vi "Main.vi"() -> ()   [LabVIEW 2019]
panel:
  out "wait mS":u16=250
  out "Board":picture
  out "Next Piece":picture
  out "Rows Cleared":u16
  out "Score":u32
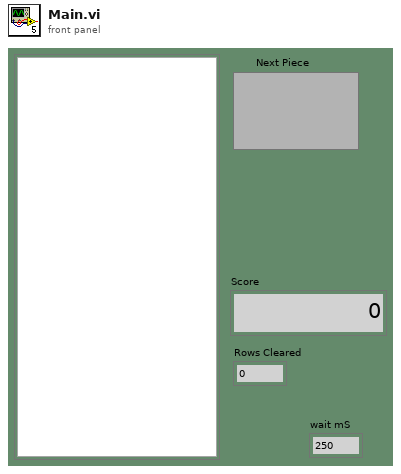
[diagram p1: front panel]
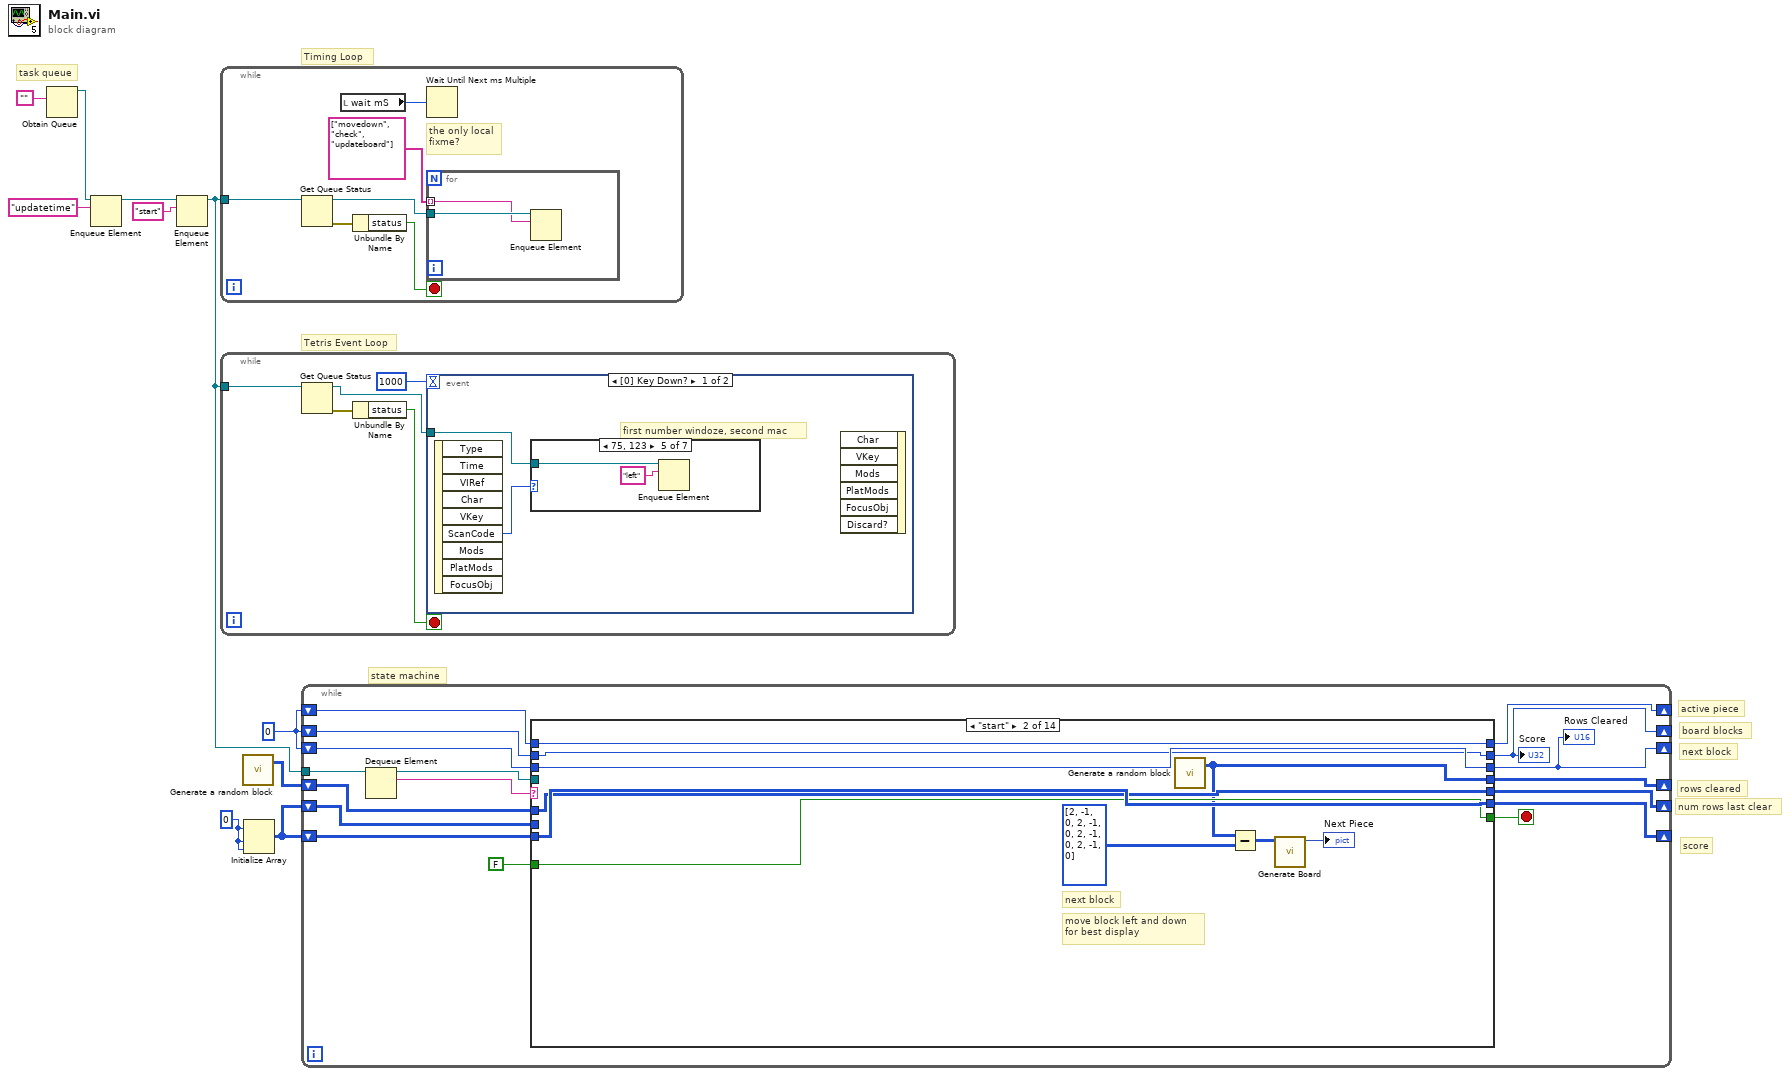
[diagram p0: block diagram]
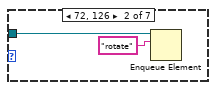
[diagram p3: hidden frame]
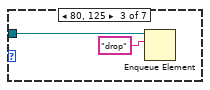
[diagram p4: hidden frame]
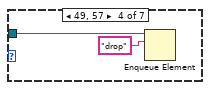
[diagram p5: hidden frame]
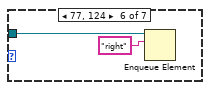
[diagram p6: hidden frame]
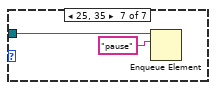
[diagram p7: hidden frame]
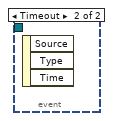
[diagram p8: hidden frame]
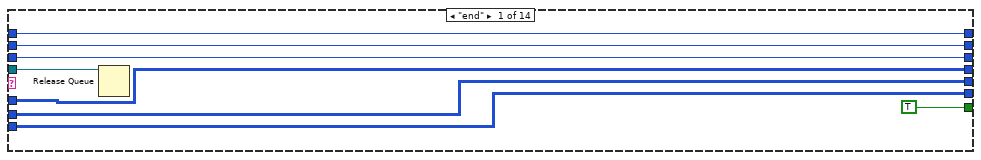
[diagram p9: hidden frame]
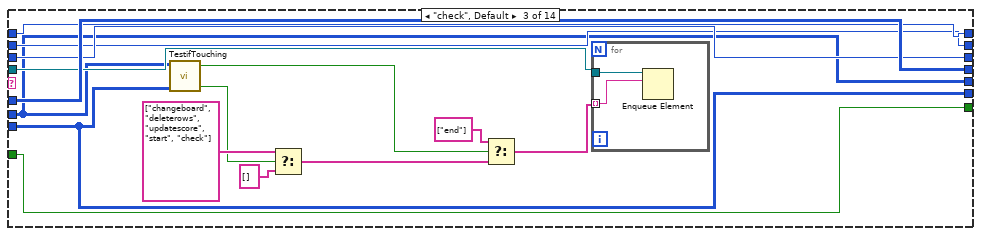
[diagram p10: hidden frame]
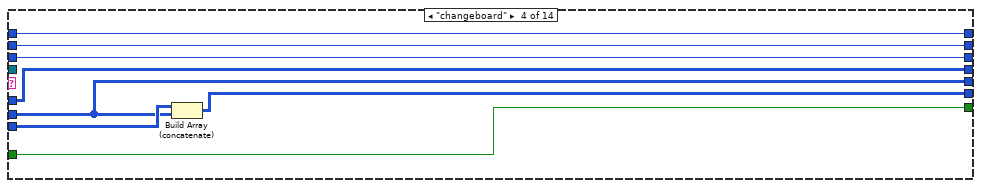
[diagram p11: hidden frame]
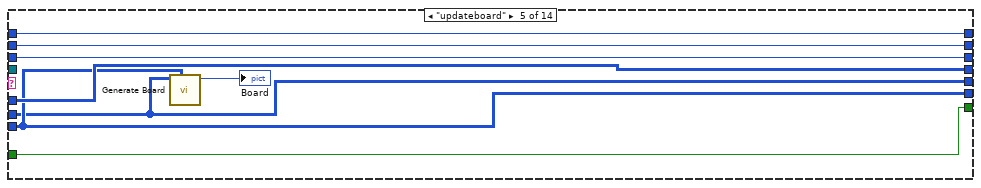
[diagram p12: hidden frame]
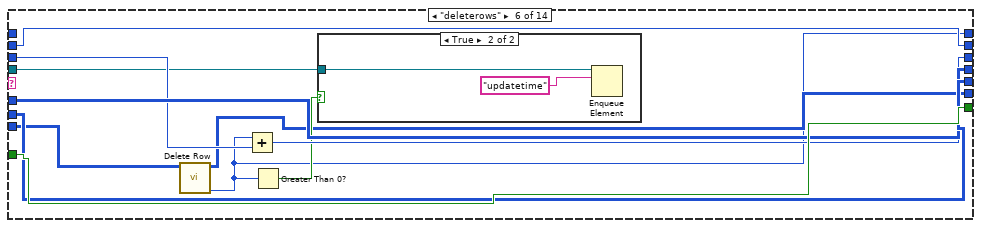
[diagram p13: hidden frame]
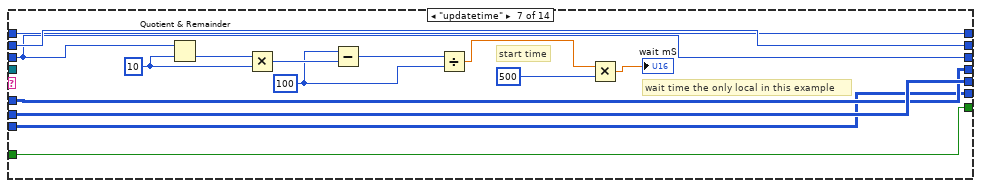
[diagram p15: hidden frame]
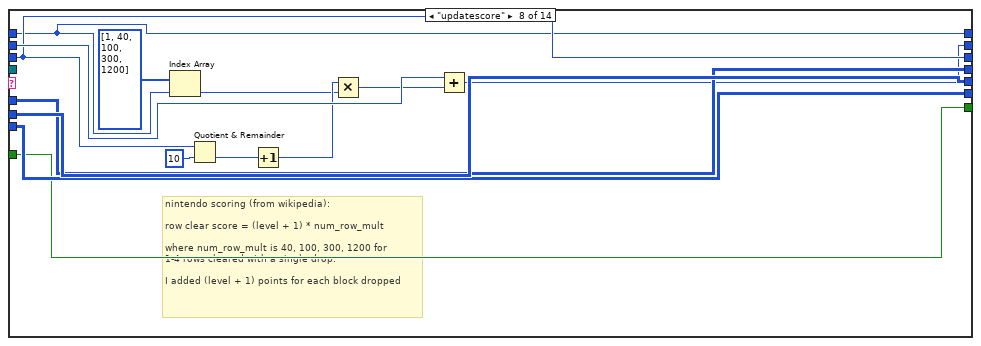
[diagram p16: hidden frame]
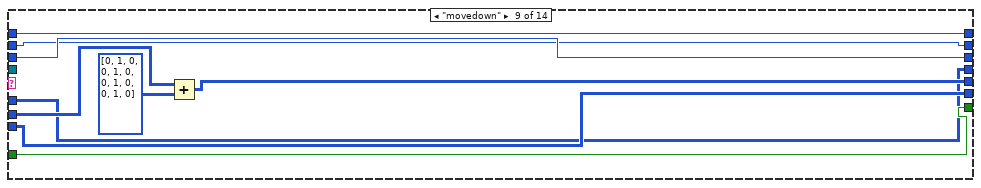
[diagram p17: hidden frame]
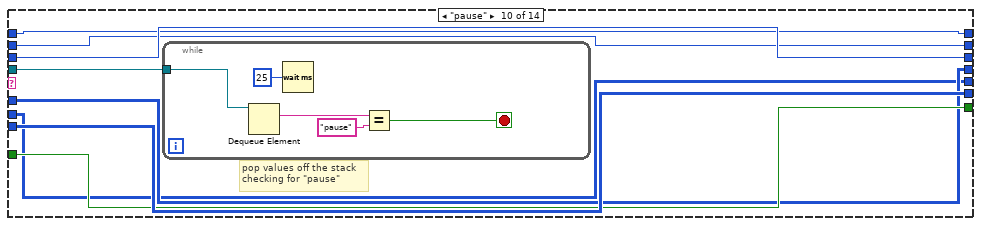
[diagram p18: hidden frame]
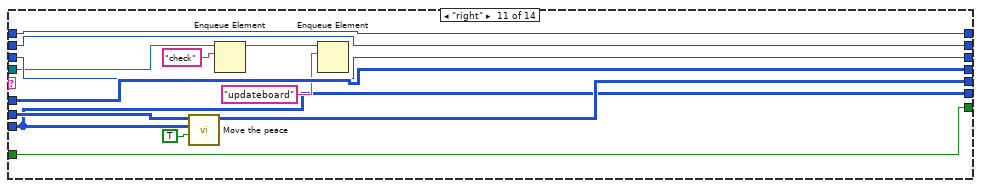
[diagram p19: hidden frame]
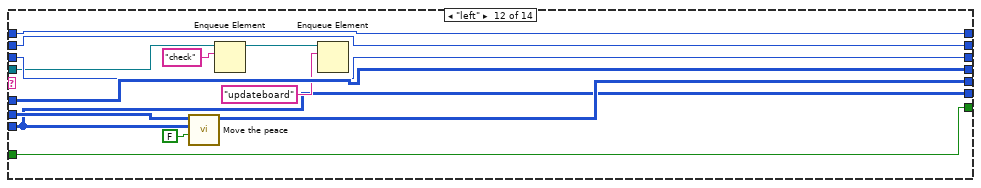
[diagram p20: hidden frame]
diagram:
  w2 = 0
  w10 = 0
  # "task queue"
  # "num rows last clear"
  # "score"
  # "rows cleared"
  # "Timing Loop"
  # "Tetris Event Loop"
  # "state machine"
  # "next block"
  # "board blocks"
  # "active piece"
  n1 = Obtain Queue(element data type="") -> (queue out=w8:refnum<queue>)  [unwired: 4 in, 2 out]
  n2 = Enqueue Element(queue=w8, element="updatetime") -> (queue out=w5:refnum<queue>)  [unwired: 2 in, 2 out]
  n3 = Enqueue Element(queue=w5, element="start") -> (queue out=w4:refnum<queue>)  [unwired: 2 in, 2 out]
  n4 = while {
    tunnel: w4 -> [w12]
    stop <- w13 stop-if-true
    # "the only local\nfixme?"
    n5 = Get Queue Status(queue=w12) -> (queue out=w11:refnum<queue>, error out=w14:errorcluster)  [unwired: 2 in, 6 out]
    n6 = local read "wait mS"() -> (w15:u16)
    n7 = Unbundle By Name(w14) -> ("status"=w13:bool)
    n8 = Wait Until Next ms Multiple(millisecond multiple=w15) -> ()  [unwired: 1 out]
    n9 = for {
      tunnel: w11 -> [w18]
      tunnel: string[] ["movedown", "check", "updateboard"] -> [w17] mode=indexing
      n10 = Enqueue Element(queue=w18, element=w17) -> ()  [unwired: 2 in, 3 out]
    }
  }
  n11 = while {
    tunnel: w4 -> [w20]
    stop <- w21 stop-if-true
    n12 = Get Queue Status(queue=w20) -> (queue out=w19:refnum<queue>, error out=w22:errorcluster)  [unwired: 2 in, 6 out]
    n13 = Unbundle By Name(w22) -> ("status"=w21:bool)
    n14 = event shown="[0] Key Down?" {
      selector: _ -> [_ _]
      dyn-events: _ -> [_ _]
      timeout: 1000 -> [_ _]
      tunnel: w19 -> [w24 _]
      event Key Down? {
        # "first number windoze, second mac"
        n15 = event-data() -> ("ScanCode"=w25:i16)  [unwired: 1 in, 8 out]
        n16 = case shown="75, 123" w25 {
          tunnel: w24 -> [_ w27 w29 w31 w33 w35 w37]
          frame 0, Default {
          }
          frame 72, 126 {
            n17 = Enqueue Element(queue=w27, element="rotate") -> ()  [unwired: 2 in, 3 out]
          }
          frame 80, 125 {
            n18 = Enqueue Element(queue=w29, element="drop") -> ()  [unwired: 2 in, 3 out]
          }
          frame 49, 57 {
            n19 = Enqueue Element(queue=w31, element="drop") -> ()  [unwired: 2 in, 3 out]
          }
          frame 75, 123 {
            n20 = Enqueue Element(queue=w33, element="left") -> ()  [unwired: 2 in, 3 out]
          }
          frame 77, 124 {
            n21 = Enqueue Element(queue=w35, element="right") -> ()  [unwired: 2 in, 3 out]
          }
          frame 25, 35 {
            n22 = Enqueue Element(queue=w37, element="pause") -> ()  [unwired: 2 in, 3 out]
          }
        }
        n23 = event-data() -> ()  [unwired: 7 in, 1 out]
      }
      event Timeout {
        n24 = event-data() -> ()  [unwired: 1 in, 3 out]
      }
    }
  }
  n25 = call "Generate a random block.vi"() -> ("Block Array"=w1:u8[][])  [unwired: 3 in]
  n26 = Initialize Array(w10, w10, w10) -> (w6:i32[][])
  n27 = while {
    shift-right: [w44] -> _
    shift-left: w6 -> [w52]
    shift-right: [w45] -> _
    shift-left: w6 -> [w51]
    shift-right: [w49] -> _
    shift-left: w1 -> [w50]
    tunnel: w4 -> [w48]
    shift-right: [w42] -> _
    shift-left: w2 -> [w43]
    shift-right: [w39] -> _
    shift-left: w2 -> [w40]
    shift-right: [w38] -> _
    shift-left: w2 -> [w41]
    stop <- w53 stop-if-true
    n28 = Dequeue Element(queue=w48) -> (queue out=w47:refnum<queue>, element=w46:string)  [unwired: 2 in, 2 out]
    n29 = case shown="\"start\"" w46 {
      tunnel: FALSE -> [_ w66 w87 w97 w105 w116 w133 w145 w152 w163 w182 w195 w207 w219]
      tunnel: [TRUE w66 w87 w97 w105 w116 w133 w145 w152 w163 w182 w195 w207 w219] -> w53
      tunnel: [w61 w71 w76 w95 w98 w115 w132 w147 w153 w161 w172 w185 w196 w210] -> w44
      tunnel: w52 -> [w61 _ w76 w95 w98 w115 w132 w147 w155 w161 w173 w186 w198 w210]
      tunnel: w51 -> [w60 w72 w75 w96 w99 w108 w130 w146 w156 w164 w171 w184 w197 w209]
      tunnel: [w60 w72 w75 w94 w99 w107 w130 w146 w156 w164 w171 w184 w197 w209] -> w45
      tunnel: w50 -> [w59 w71 w85 w93 w104 w114 w131 w144 w151 w162 w181 w194 w206 w218]
      tunnel: [w59 w65 w85 w93 w104 w114 w131 w144 w151 w162 w181 w194 w206 w218] -> w49
      tunnel: w47 -> [w55 _ w84 _ _ w111 _ _ _ w160 w176 w189 w199 w215]
      tunnel: [w58 w69 w79 w92 w103 w112 w128 w141 w150 w159 w180 w193 w205 w213] -> w42
      tunnel: w43 -> [w58 w69 w79 w92 w103 w113 w128 w141 w150 w159 w180 w193 w205 w213]
      tunnel: [w57 w68 w78 w91 w102 w106 w127 w139 w149 w158 w179 w192 w204 w212] -> w39
      tunnel: [w56 w67 w77 w90 w101 w110 w129 w135 w148 w157 w178 w191 w203 w211] -> w38
      tunnel: w41 -> [w56 w67 w77 w90 w101 w110 w129 w143 w148 w157 w178 w191 w203 w211]
      tunnel: w40 -> [w57 w68 w78 w91 w102 _ w127 w139 w149 w158 w179 w192 w204 w212]
      frame "end" {
        n30 = Release Queue(queue=w55) -> ()  [unwired: 2 in, 3 out]
      }
      frame "start" {
        # "move block left and down\nfor best display"
        # "next block"
        n31 = call "Generate a random block.vi"() -> ("Block Array"=w65:u8[][])  [unwired: 3 in]
        n32 = Subtract(x=w65, y=i32[][] [[2, -1, 0], [2, -1, 0], [2, -1, 0], [2, -1, 0]]) -> (x-y=w63:i32[][])
        n33 = call "Generate Board.vi"("Piece Array"=w63) -> ("Picture"=→"Next Piece":picture)  [unwired: 10 in]
      }
      frame "check", Default {
        n34 = call "TestifTouching.vi"("Piece Array"=w76, "board array"=w75) -> ("Lost"=w74:bool, "Touching"=w73:bool)  [unwired: 4 in, 1 out]
        n35 = Select(t=string[] ["changeboard", "deleterows", "updatescore", "start", "check"], s=w73, f=string[] []) -> (s? t:f=w86:string[])
        n36 = Select(t=string[] ["end"], s=w74, f=w86) -> (s? t:f=w83:string[])
        n37 = for {
          tunnel: w84 -> [w89]
          tunnel: w83 -> [w88] mode=indexing
          n38 = Enqueue Element(queue=w89, element=w88) -> ()  [unwired: 2 in, 3 out]
        }
      }
      frame "changeboard" {
        n39 = Build Array (concatenate)(w96, w95) -> (w94:i32[][])
      }
      frame "updateboard" {
        n40 = call "Generate Board.vi"("Board Array"=w99, "Piece Array"=w98) -> ("Picture"=→"Board":picture)  [unwired: 9 in]
      }
      frame "deleterows" {
        n41 = call "Delete Row.vi"("board array in"=w108) -> ("Rows Deleted"=w106:u16, "board array out"=w107:u8[][])  [unwired: 9 in]
        n42 = Add(x=w106, y=w113) -> (x+y=w112:i32)
        n43 = Greater Than 0?(x=w106) -> (x > 0?=w109:bool)
        n44 = case shown="True" w109 {
          tunnel: w111 -> [_ w117]
          frame False {
          }
          frame True {
            n45 = Enqueue Element(queue=w117, element="updatetime") -> ()  [unwired: 2 in, 3 out]
          }
        }
      }
      frame "updatetime" {
        w122 = 100
        w125 = 10
        # "start time"
        # "wait time the only local in this example"
        n46 = Quotient & Remainder(x=w128, y=w125) -> (floor(x/y)=w126:i32)  [unwired: 1 out]
        n47 = Multiply(x=w126, y=w125) -> (x*y=w124:i32)
        n48 = Subtract(x=w122, y=w124) -> (x-y=w123:i32)
        n49 = Divide(x=w123, y=w122) -> (x/y=w121:dbl)
        n50 = Multiply(x=w121, y=500) -> (x*y=→"wait mS":dbl)
      }
      frame "updatescore" {
        # "nintendo scoring (from wikipedia):\n\nrow clear score = (level + 1) * num_row_mult\n\nwhere num_row_mult is 40, 100, 300, 1200 for \n1-4 rows cleared with a single drop.\n\nI added (level + 1) points for each block dropped"
        n51 = Index Array(array=i32[] [1, 40, 100, 300, 1200], index=w139) -> (element=w136:i32)
        n52 = Quotient & Remainder(x=w141, y=10) -> (floor(x/y)=w140:i32)  [unwired: 1 out]
        n53 = Increment(x=w140) -> (x+1=w137:i32)
        n54 = Multiply(x=w137, y=w136) -> (x*y=w134:i32)
        n55 = Add(x=w143, y=w134) -> (x+y=w135:i32)
      }
      frame "movedown" {
        n56 = Add(x=w155, y=i32[][] [[0, 1, 0], [0, 1, 0], [0, 1, 0], [0, 1, 0]]) -> (x+y=w153:i32[][])
      }
      frame "pause" {
        # "pop values off the stack\nchecking for \"pause\""
        n57 = while {
          tunnel: w160 -> [w169]
          stop <- w166 stop-if-true
          n58 = Dequeue Element(queue=w169) -> (element=w167:string)  [unwired: 2 in, 3 out]
          n59 = Wait (ms)(milliseconds to wait=25) -> ()  [unwired: 1 out]
          n60 = Equal?(x=w167, y="pause") -> (x = y?=w166:bool)
        }
      }
      frame "right" {
        n61 = call "Move the peace.vi"("Move Right"=TRUE, "Stack Array"=w171, "Piece Array"=w173) -> ("Moved Piece Array"=w172:u8[][])  [unwired: 8 in]
        n62 = Enqueue Element(queue=w176, element="check") -> (queue out=w174:refnum<queue>)  [unwired: 2 in, 2 out]
        n63 = Enqueue Element(queue=w174, element="updateboard") -> ()  [unwired: 2 in, 3 out]
      }
      frame "left" {
        n64 = call "Move the peace.vi"("Move Right"=FALSE, "Stack Array"=w184, "Piece Array"=w186) -> ("Moved Piece Array"=w185:u8[][])  [unwired: 8 in]
        n65 = Enqueue Element(queue=w189, element="check") -> (queue out=w188:refnum<queue>)  [unwired: 2 in, 2 out]
        n66 = Enqueue Element(queue=w188, element="updateboard") -> ()  [unwired: 2 in, 3 out]
      }
      frame "rotate" {
        n67 = call "Rotate piece 2.vi"("Piece Array"=w198, "Stack Array"=w197) -> ("Rotated Piece Array"=w196:u8[][])  [unwired: 7 in]
        n68 = Enqueue Element(queue=w199, element="check") -> (queue out=w201:refnum<queue>)  [unwired: 2 in, 2 out]
        n69 = Enqueue Element(queue=w201, element="updateboard") -> ()  [unwired: 2 in, 3 out]
      }
      frame "drop" {
        n70 = call "TestifTouching.vi"("Piece Array"=w210, "board array"=w209) -> ("min Distance"=w208:i16)  [unwired: 4 in, 2 out]
        n71 = for {
          N: w208 -> [_]
          tunnel: ["movedown"] -> w217 mode=indexing
        }
        n72 = Build Array (concatenate)(w217, "check") -> (w214:string[])
        n73 = for {
          tunnel: w215 -> [w221]
          tunnel: w214 -> [w220] mode=indexing
          n74 = Enqueue Element(queue=w221, element=w220) -> ()  [unwired: 2 in, 3 out]
        }
      }
    }
    "Rows Cleared" <- w42
    "Score" <- w38
  }
